vi "Init.vi"(8 "error in (no error)":errorcluster, 10 "Shutdown Event":refnum<user-event>, 11 "Modbus in":refnum<class "Modbus.lvclass">) -> (0 "error out":errorcluster, 3 "Modbus out":refnum<class "Modbus.lvclass">)   [LabVIEW 2020, in "Modbus.lvlib" / "Modbus.lvclass"]
uses:
  Modbus.lvclass
  Plugin Interfaces/Controller Interface/Controller Interface.lvlibp/Controller Interface Class/Controller Interface.lvclass
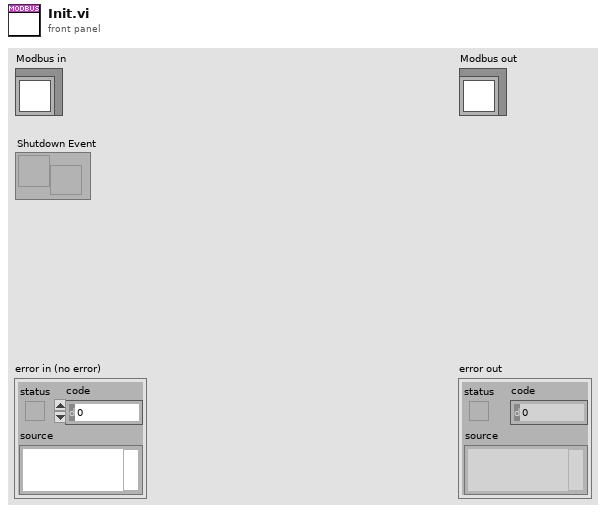
[diagram p1: front panel]
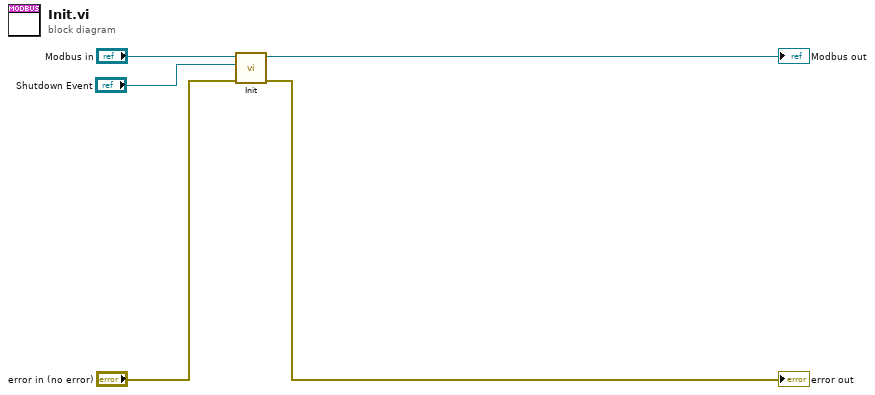
[diagram p0: block diagram]
diagram:
  n1 = call-parent "Init.vi"("error in (no error)"="error in (no error)", "Shutdown Event"="Shutdown Event", "Controller Interface in"="Modbus in") -> ("error out"=→"error out":errorcluster, "Controller Interface out"=→"Modbus out":refnum<class "Modbus.lvclass">)  [unwired: 7 in]
